vi "form voltage alarm string.vi"(0 "Xmon":dbl[][](array[numeric]), 1 "Xset":dbl[][](array[numeric]), 2 "Timestamps":dbl[][](array[numeric]), 3 "Alarm Tolerance (frac)":dbl=0.2 format="%#_13g", 4 "Warning Tolerance (frac)":dbl=0.1 format="%#_13g", 5 "error in":errorcluster, 6 "Alarm:T Warning:F":bool, 7 "Crate Enable":bool, 8 "Current:T Voltage:F":bool, 10 "Num Channels Read":i32, 12 "Start index":i32) -> (14 "Error Status String":string, 15 "All channels in error":string, 16 "Error Logged":bool[](array[boolean]), 17 "Error Array":string[][](array[string]), 18 "Status Strings":string[](array[string]), 19 "Error Out":errorcluster)   [LabVIEW 2018]
uses:
  channel_cluster.ctl
  CAEN globals.vi
  <userlib>/_OpenG.lib/array/array.llb/Search 1D Array (Boolean)__ogtk.vi
  <userlib>/_OpenG.lib/array/array.llb/Index 1D Array Elements (DBL)__ogtk.vi
  <userlib>/_OpenG.lib/array/array.llb/Index 1D Array Elements (Boolean)__ogtk.vi
  <userlib>/_OpenG.lib/array/array.llb/Index 1D Array Elements (String)__ogtk.vi
panel:
  in  "Channel Array Val":T1[](array[typedef]) {"Vfile (V)" format="%.1f V"}
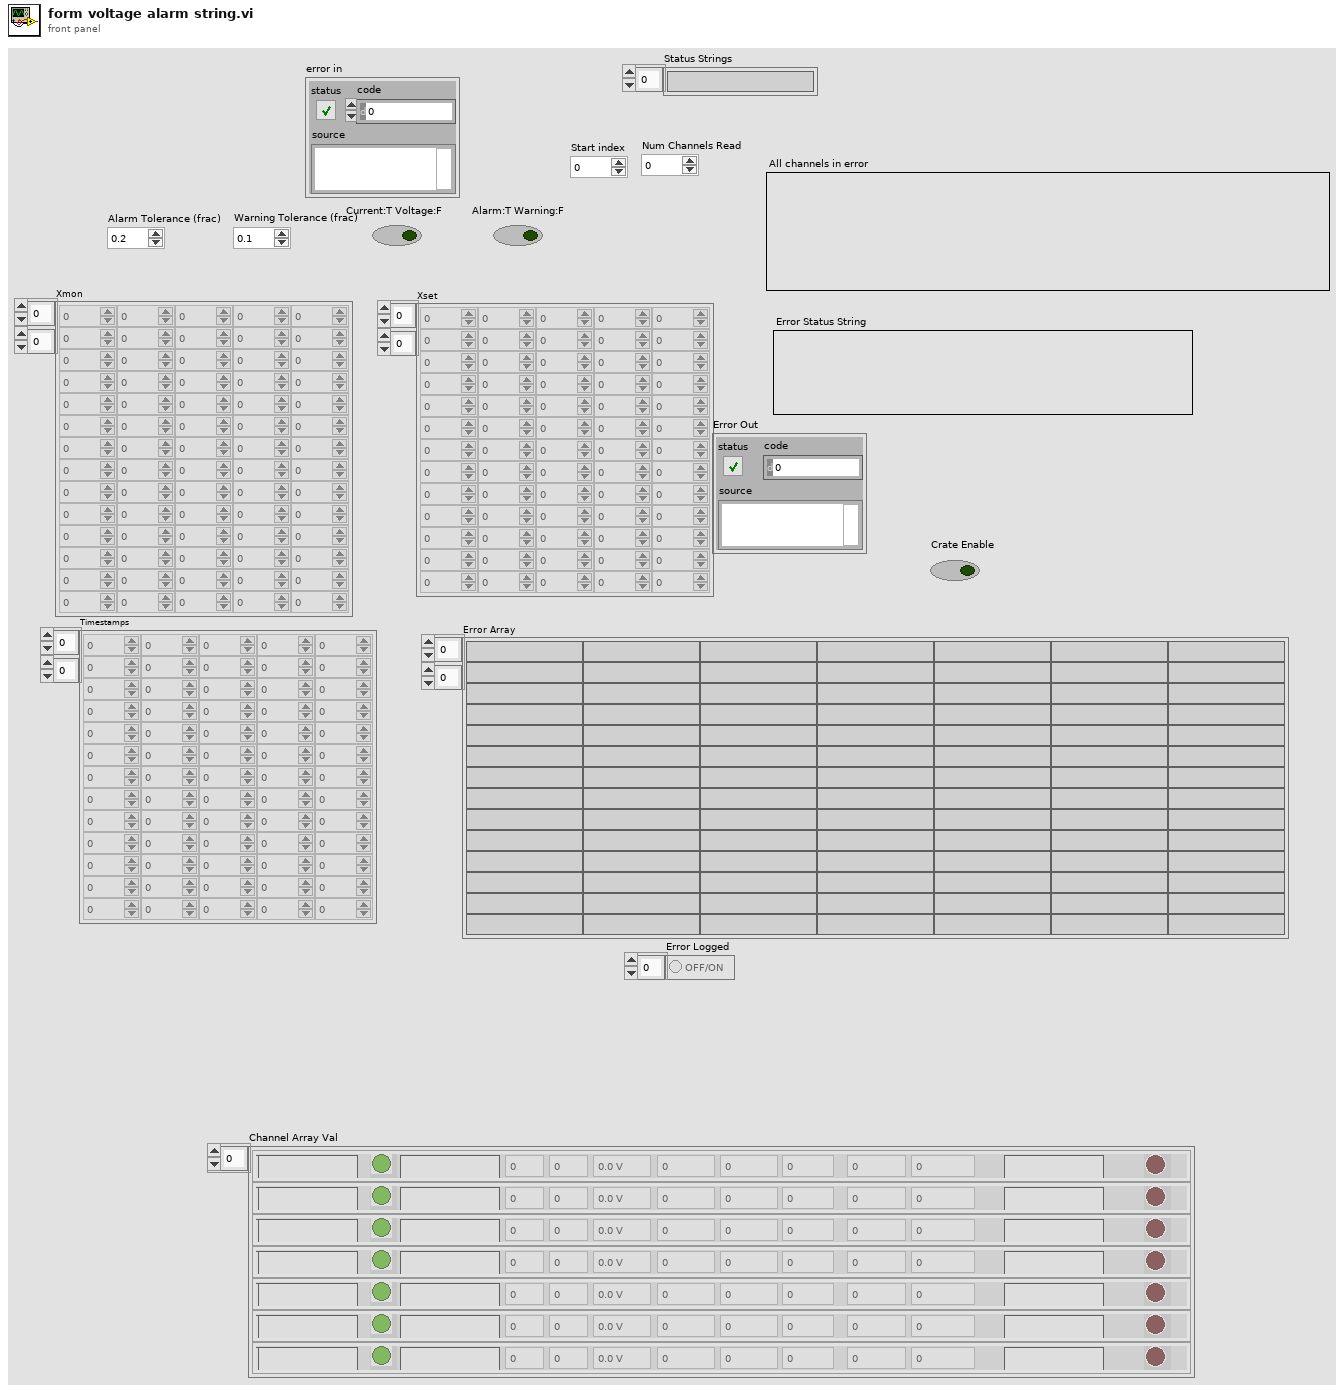
[diagram p1: front panel]
types:
  T1 = typedef "channel_cluster.ctl" = cluster{"Channel Name":string, "Crate":i32, "Card Type":string, "Card":i32, "Channel":i32, "Status Icon":picture, "Vmon (V)":dbl, "Vset (V)":dbl, "Imon (A)":dbl, "Iset (A)":dbl, "Timestamp":string, "ON/OFF":bool, "Status":string, "Vswmax (V)":dbl, "Flag":bool, "Vfile (V)":dbl, "Error Logged":bool[], "enable_file":bool}
  T2 = cluster{"Crate num":i32, "Slot nums":i32[], "Channel nums":i32[][], "N chans":i32[]}[]
  T3 = cluster{"Numeric":i32, "Indices of Elements":i32[], "Indices of Elements":i32[][], "Indices of Elements":i32[]}
  T4 = cluster{"Numeric":i32, "Indices of Elements":i32[], "Indices of Elements":i32[][], "Indices of Elements":i32[]}[]
  T5 = cluster{"Numeric":i32, "Indices of Elements":i32[], i32[][], i32[]}
  T6 = cluster{"Numeric":i32, "Indices of Elements":i32[], "Channel nums":i32[][], "N chans":i32[]}[]
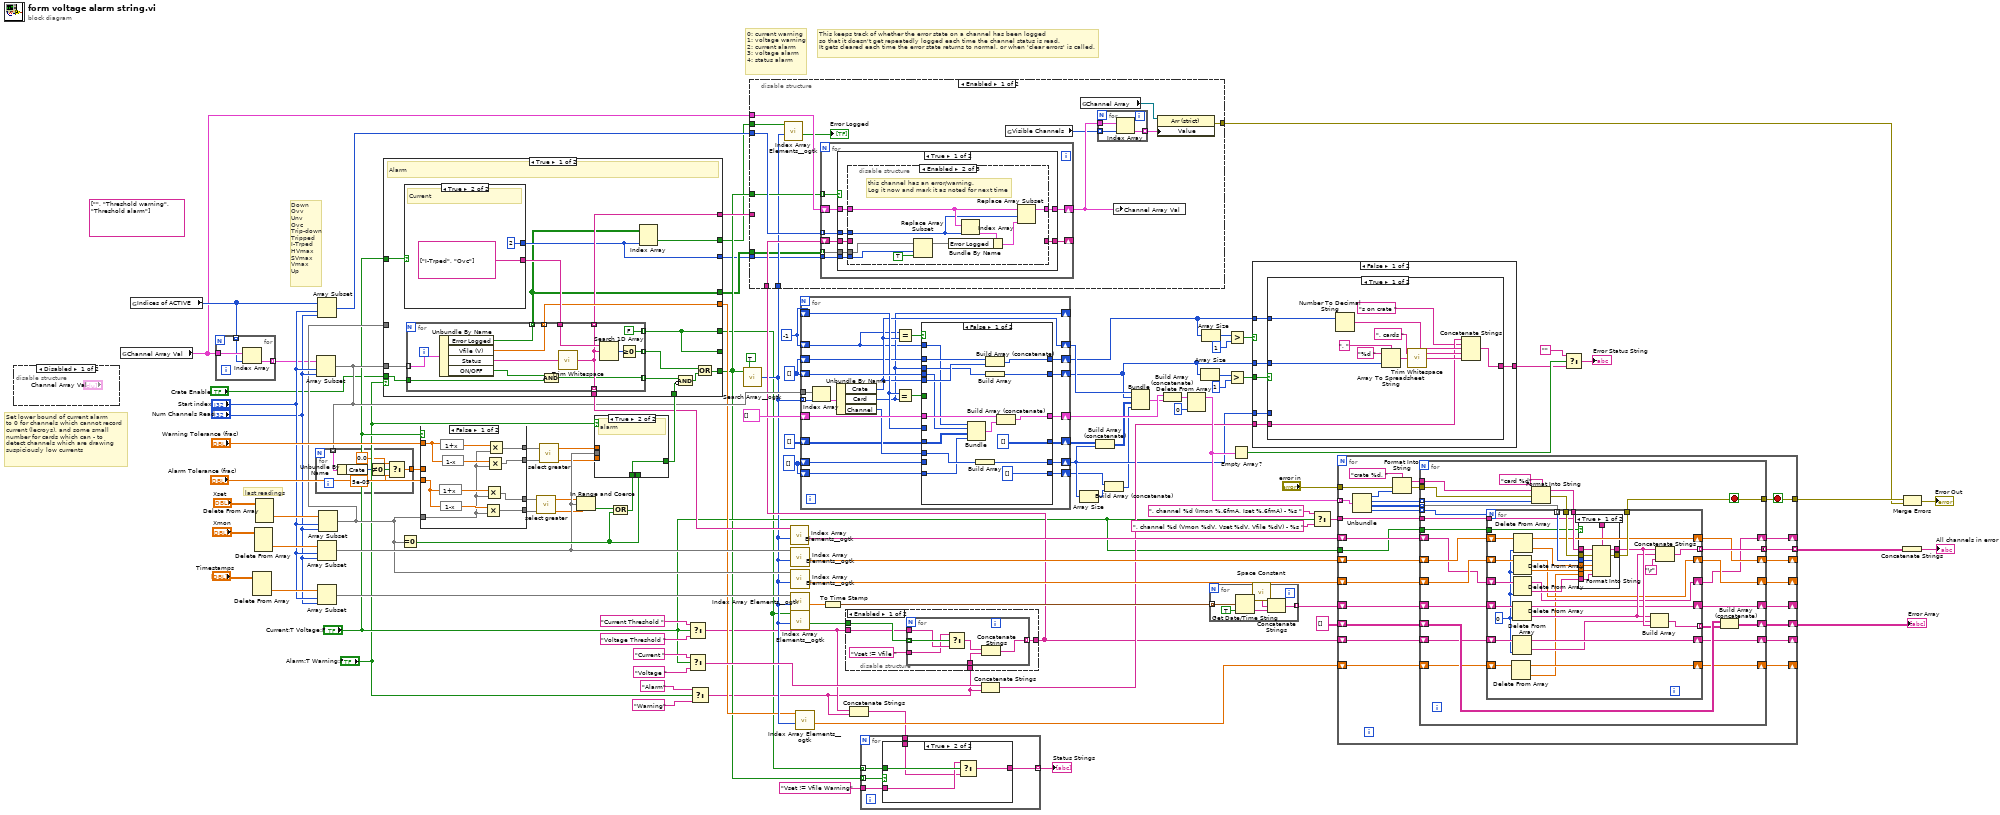
[diagram p0: block diagram]
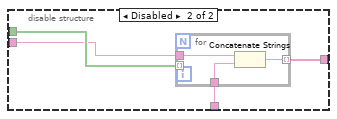
[diagram p2: hidden frame]
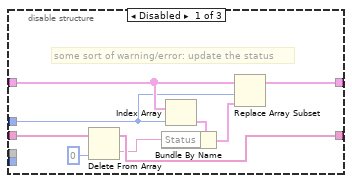
[diagram p3: hidden frame]
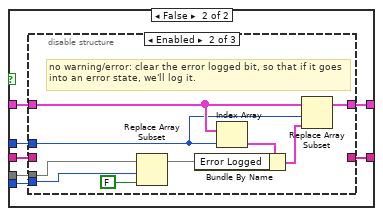
[diagram p5: hidden frame]
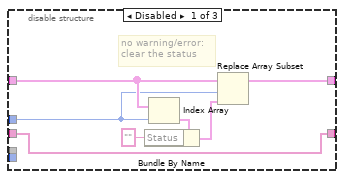
[diagram p6: hidden frame]
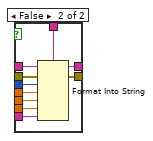
[diagram p11: hidden frame]
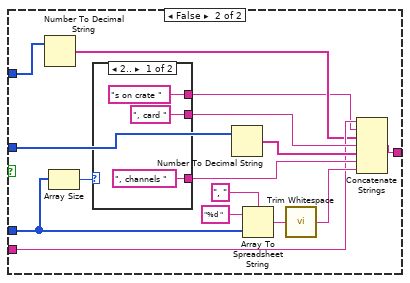
[diagram p12: hidden frame]
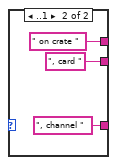
[diagram p13: hidden frame]
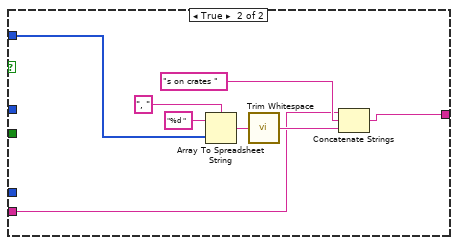
[diagram p14: hidden frame]
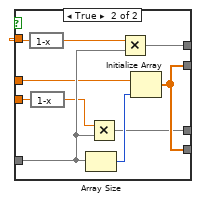
[diagram p15: hidden frame]
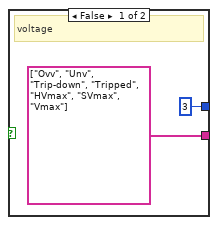
[diagram p16: hidden frame]
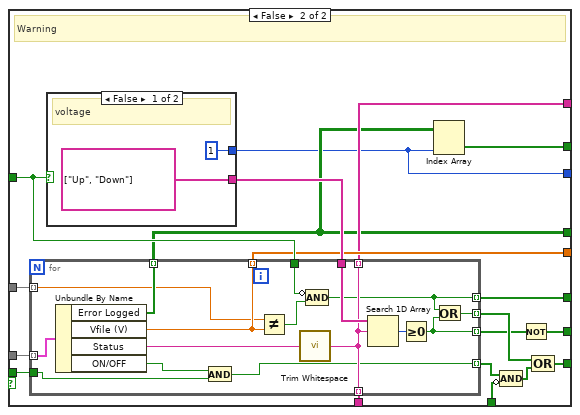
[diagram p17: hidden frame]
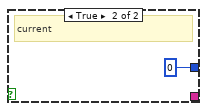
[diagram p18: hidden frame]
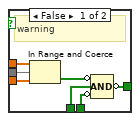
[diagram p19: hidden frame]
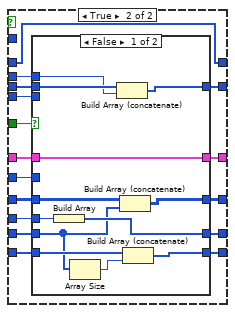
[diagram p20: hidden frame]
diagram:
  w33 = i32[] [] ("Indices of Elements")
  (unwired) string[] ["", "Threshold warning", "Threshold alarm"] ("items to filter")
  w45 = i32[] [] ("Indices of Elements")
  w46 = -1 ("Numeric")
  # "0: current warning\n1: voltage warning\n2: current alarm\n3: voltage alarm\n4: status alarm"
  # "This keeps track of whether the error state on a channel has been logged\nso that it doesn't get repeatedly logged each time the channel status is read.\nIt gets cleared each time the error state returns to normal, or when 'clear errors' is called."
  # "Set lower bound of current alarm\nto 0 for channels which cannot record\ncurrent (lecroys), and some small\nnumber for cards which can - to\ndetect channels which are drawing\nsuspiciously low currents"
  # "Down\nOvv\nUnv\nOvc\nTrip-down\nTripped\nI-Trped\nHVmax\nSVmax\nVmax\nUp"
  # "last readings"
  n1 = disable-structure shown="Disabled" {
    frame Disabled {
    }
    frame Enabled {
    }
  }
  n2 = global read "CAEN globals.vi" "Channel Array Val"() -> (w34:T1[])
  n3 = global read "CAEN globals.vi" "Indices of ACTIVE"() -> (w57:i32[])
  n4 = for {
    tunnel: w34 -> [w109]
    tunnel: [w108] -> w23 mode=indexing
    tunnel: w57 -> [w107] mode=indexing
    n5 = Index Array(array=w109, index=w107) -> (element=w108:T1)
  }
  n6 = Delete From Array(array="Timestamps") -> (deleted portion=w59:dbl[])  [unwired: 3 in, 1 out]
  n7 = Delete From Array(array="Xmon") -> (deleted portion=w61:dbl[])  [unwired: 3 in, 1 out]
  n8 = Delete From Array(array="Xset") -> (deleted portion=w62:dbl[])  [unwired: 3 in, 1 out]
  n9 = Array Subset(array=w23, index="Start index", length="Num Channels Read") -> (w52:T1[])
  n10 = for {
    tunnel: w52 -> [w115] mode=indexing
    tunnel: [w110] -> w51
    n11 = Unbundle By Name(w115) -> ("Crate"=w114:i32)
    n12 = Not Equal To 0?(x=w114) -> (x != 0?=w113:bool)
    n13 = Select(t=0.0 ("element"), s=w113, f=5e-05 ("element")) -> (s? t:f=w110:dbl)
  }
  n14 = Array Subset(array=w57, index="Start index", length="Num Channels Read") -> (w22:i32[])
  n15 = Array Subset(array=w61, index="Start index", length="Num Channels Read") -> (w60:dbl[])
  n16 = Array Subset(array=w59, index="Start index", length="Num Channels Read") -> (w58:dbl[])
  n17 = Array Subset(array=w62, index="Start index", length="Num Channels Read") -> (w35:dbl[])
  n18 = Equal To 0?(x=w35) -> (x = 0?=w72:bool[])
  n19 = case shown="False" "Current:T Voltage:F" {
    tunnel: [w118 w135] -> w11
    tunnel: [w119 w127] -> w14
    tunnel: [w124 w132] -> w10
    tunnel: [w122 w135] -> w9
    tunnel: "Warning Tolerance (frac)" -> [w126 w133]
    tunnel: "Alarm Tolerance (frac)" -> [w117 w131]
    tunnel: w35 -> [w116 w134]
    tunnel: w51 -> [_ w128]
    frame False {
      n20 = expression code="1+x"(w117) -> (w120:dbl)
      n21 = expression code="1+x"(w126) -> (w125:dbl)
      n22 = expression code="1-x"(w117) -> (w121:dbl)
      n23 = expression code="1-x"(w126) -> (w123:dbl)
      n24 = Multiply(x=w121, y=w116) -> (x*y=w118:dbl[])
      n25 = Multiply(x=w120, y=w116) -> (x*y=w119:dbl[])
      n26 = Multiply(x=w123, y=w116) -> (x*y=w122:dbl[])
      n27 = Multiply(x=w125, y=w116) -> (x*y=w124:dbl[])
    }
    frame True {
      n28 = expression code="1-x"(w133) -> (w130:dbl)
      n29 = expression code="1-x"(w131) -> (w129:dbl)
      n30 = Array Size(array=w134) -> (size(s)=w136:i32)
      n31 = Multiply(x=w129, y=w134) -> (x*y=w127:dbl[])
      n32 = Multiply(x=w130, y=w134) -> (x*y=w132:dbl[])
      n33 = Initialize Array(w128, w136) -> (w135:dbl[])
    }
  }
  n34 = call "select greater.vi"("Array 1 in"=w14, "Array 2 in"=w11) -> ("Array of higher vals"=w13:dbl[], "Array of lower vals"=w12:dbl[])  [unwired: 24 in]
  n35 = call "select greater.vi"("Array 1 in"=w10, "Array 2 in"=w9) -> ("Array of higher vals"=w7:dbl[], "Array of lower vals"=w8:dbl[])  [unwired: 24 in]
  n36 = In Range and Coerce(upper limit=w13, x=w60, lower limit=w12) -> (In Range?=w54:bool[])  [unwired: 1 out]
  n37 = Compound Arithmetic op=OR(w54, w72) -> (w65:bool[])
  n38 = case shown="True" "Alarm:T Warning:F" {
    tunnel: w60 -> [w143 _]
    tunnel: w65 -> [w137 w144]
    tunnel: [w141 w144] -> w74
    tunnel: w72 -> [w138 _]
    tunnel: w7 -> [w140 _]
    tunnel: w8 -> [w139 _]
    frame False {
      # "warning"
      n39 = In Range and Coerce(upper limit=w140, x=w143, lower limit=w139) -> (In Range?=w142:bool[])  [unwired: 1 out]
      n40 = Compound Arithmetic op=AND(invert w142, w137, invert w138) -> (invert w141:bool[])
    }
    frame True {
      # "alarm"
    }
  }
  n41 = case shown="True" "Alarm:T Warning:F" {
    tunnel: [w157 w192] -> w20
    tunnel: w74 -> [w156 w191]
    tunnel: [w160 w195] -> w73
    tunnel: [w151 w184] -> w21
    tunnel: w52 -> [w159 w194]
    tunnel: "Current:T Voltage:F" -> [w153 w186]
    tunnel: [w145 w179] -> _
    tunnel: w35 -> [_ w187]
    tunnel: [w152 w185] -> w26
    tunnel: [w150 w183] -> w6
    tunnel: [w148 w182] -> w5
    tunnel: [w149 w181] -> w4
    tunnel: "Crate Enable" -> [w146 w178]
    tunnel: [w145 w177] -> w1
    frame True {
      # "Alarm"
      n42 = case shown="True" w153 {
        tunnel: [string[] ["Ovv", "Unv", "Trip-down", "Tripped", "HVmax", "SVmax", "Vmax"] ("items to filter") string[] ["I-Trped", "Ovc"] ("items to filter")] -> w154
        tunnel: [3 2] -> w149
        frame False {
          # "voltage"
        }
        frame True {
          # "Current"
        }
      }
      n43 = for {
        tunnel: w159 -> [w176] mode=indexing
        tunnel: [w171] -> w158 mode=indexing
        tunnel: w154 -> [w174]
        tunnel: [w172] -> w160 mode=indexing
        tunnel: [w172] -> w151 mode=indexing
        tunnel: [FALSE ("Element Data")] -> w145 mode=indexing
        tunnel: [w169] -> w152 mode=indexing
        tunnel: [w168] -> w148 mode=indexing
        tunnel: [w166] -> w147 mode=indexing
        tunnel: w146 -> [w165]
        n44 = Unbundle By Name(w176) -> ("Error Logged"=w168:bool[], "Vfile (V)"=w169:dbl, "Status"=w173:string, "ON/OFF"=w167:bool)
        n45 = And(x=w167, y=w165) -> (x .and. y?=w166:bool)
        n46 = call <vilib>:"Trim Whitespace.vi"("string"=w173) -> ("trimmed string"=w172:string)  [unwired: 1 in]
        n47 = Search 1D Array(1D array=w174, element=w172) -> (index of element=w175:i32)  [unwired: 1 in]
        n48 = Greater Or Equal To 0?(x=w175) -> (x >= 0?=w171:bool)
      }
      n49 = Index Array(array=w148, index (col)=w149) -> (element=w150:bool[])  [unwired: 1 in]
      n50 = Compound Arithmetic op=AND(w147, invert w156) -> (w155:bool[])
      n51 = Compound Arithmetic op=OR(w158, w155) -> (w157:bool[])
    }
    frame False {
      # "Warning"
      n52 = case shown="False" w186 {
        tunnel: [string[] ["Up", "Down"] ("items to filter") _] -> w188
        tunnel: [1 0] -> w181
        frame False {
          # "voltage"
        }
        frame True {
          # "current"
        }
      }
      n53 = for {
        tunnel: w194 -> [w214] mode=indexing
        tunnel: [w201] -> w190 mode=indexing
        tunnel: [w205] -> w193 mode=indexing
        tunnel: w188 -> [w212]
        tunnel: [w210] -> w195 mode=indexing
        tunnel: [w210] -> w184 mode=indexing
        tunnel: w187 -> [w203] mode=indexing
        tunnel: w186 -> [w208]
        tunnel: [w207] -> w185 mode=indexing
        tunnel: [w206] -> w182 mode=indexing
        tunnel: [w204] -> w180 mode=indexing
        tunnel: w178 -> [w200]
        tunnel: [w199] -> w177 mode=indexing
        n54 = Unbundle By Name(w214) -> ("Error Logged"=w206:bool[], "Vfile (V)"=w207:dbl, "Status"=w211:string, "ON/OFF"=w202:bool)
        n55 = And(x=w202, y=w200) -> (x .and. y?=w201:bool)
        n56 = Not Equal?(x=w203, y=w207) -> (x != y?=w209:bool)
        n57 = call <vilib>:"Trim Whitespace.vi"("string"=w211) -> ("trimmed string"=w210:string)  [unwired: 1 in]
        n58 = Compound Arithmetic op=AND(invert w208, w209) -> (w199:bool)
        n59 = Search 1D Array(1D array=w212, element=w210) -> (index of element=w213:i32)  [unwired: 1 in]
        n60 = Greater Or Equal To 0?(x=w213) -> (x >= 0?=w204:bool)
        n61 = Or(x=w199, y=w204) -> (x .or. y?=w205:bool)
      }
      n62 = Index Array(array=w182, index (col)=w181) -> (element=w183:bool[])  [unwired: 1 in]
      n63 = Compound Arithmetic op=AND(w190, invert w191) -> (w189:bool[])
      n64 = Not(x=w180) -> (.not. x?=w179:bool[])
      n65 = Compound Arithmetic op=OR(w193, w189) -> (w192:bool[])
    }
  }
  n66 = Select(t="Current Threshold " ("Card type"), s="Current:T Voltage:F", f="Voltage Threshold " ("Card type")) -> (s? t:f=w18:string)
  n67 = Select(t="Current " ("Card type"), s="Current:T Voltage:F", f="Voltage " ("Card type")) -> (s? t:f=w47:string)
  n68 = Select(t="Alarm" ("Card type"), s="Alarm:T Warning:F", f="Warning" ("Card type")) -> (s? t:f=w17:string)
  n69 = call-poly <userlib>:"Search Array__ogtk.vi"("Array"=w20, "Element Data"=TRUE) -> ("Indices of Elements"=w27:i32[])  [unwired: 7 in]
  n70 = call-poly <userlib>:"Index Array Elements__ogtk.vi"("indices"=w27, "array"=w73) -> ("elements"=w55:string[])  [unwired: 9 in]
  n71 = call-poly <userlib>:"Index Array Elements__ogtk.vi"("indices"=w27, "array"=w60) -> ("elements"=w80:dbl[])  [unwired: 9 in]
  n72 = call-poly <userlib>:"Index Array Elements__ogtk.vi"("indices"=w27, "array"=w35) -> ("elements"=w79:dbl[])  [unwired: 9 in]
  n73 = call-poly <userlib>:"Index Array Elements__ogtk.vi"("indices"=w27, "array"=w58) -> ("elements"=w75:dbl[])  [unwired: 9 in]
  n74 = call-poly <userlib>:"Index Array Elements__ogtk.vi"("indices"=w27, "array"=w1) -> ("elements"=w28:bool[])  [unwired: 9 in]
  n75 = call-poly <userlib>:"Index Array Elements__ogtk.vi"("indices"=w27, "array"=w26) -> ("elements"=w25:dbl[])  [unwired: 9 in]
  n76 = for {
    tunnel: w27 -> [w231] mode=indexing
    shift-right: [w221] -> _
    shift-left: w46 -> [w227]
    shift-right: [w236] -> w40
    shift-left: i32[][] [] ("Indices of Elements") -> [w217]
    shift-right: [w235] -> w91
    shift-left: T2 [] -> [w234]
    shift-right: [w232] -> w37
    shift-left: w45 -> [w233]
    tunnel: w52 -> [w230]
    shift-right: [w224] -> w42
    shift-left: w46 -> [w220]
    shift-right: [w222] -> w38
    shift-left: w45 -> [w223]
    shift-right: [w218] -> w32
    shift-left: w33 -> [w219]
    shift-right: [w215] -> w30
    shift-left: w33 -> [w216]
    n77 = Index Array(array=w230, index=w231) -> (element=w229:T1)
    n78 = Unbundle By Name(w229) -> ("Crate"=w224:i32, "Card"=w221:i32, "Channel"=w228:i32)
    n79 = Equal?(x=w227, y=w221) -> (x = y?=w225:bool)
    n80 = Equal?(x=w220, y=w224) -> (x = y?=w226:bool)
    n81 = case shown="False" w226 {
      tunnel: w217 -> [w241 w268]
      tunnel: [i32[][] [] ("Indices of Elements") w267] -> w236
      tunnel: [w248 w266] -> w235
      tunnel: w234 -> [w249 w265]
      tunnel: w233 -> [w242 w264]
      tunnel: [w244 w263] -> w232
      tunnel: w228 -> [w246 w262]
      tunnel: w227 -> [_ w261]
      tunnel: w225 -> [_ w260]
      tunnel: w224 -> [w247 w259]
      tunnel: w223 -> [w252 w258]
      tunnel: [w251 w258] -> w222
      tunnel: w221 -> [w245 w255]
      tunnel: w220 -> [w243 _]
      tunnel: w219 -> [_ w256]
      tunnel: [w240 w257] -> w218
      tunnel: w216 -> [w238 w254]
      tunnel: [i32[] [] ("Indices of Elements") w253] -> w215
      frame False {
        n82 = Bundle("Numeric"=w243, "Indices of Elements"=w242, "Indices of Elements"=w241, "Indices of Elements"=w238) -> (w250:T3)  [unwired: 1 in]
        n83 = Build Array(w246) -> (w240:i32[])
        n84 = Build Array (concatenate)(w252, w247) -> (w251:i32[])
        n85 = Build Array(w245) -> (w244:i32[])
        n86 = Build Array (concatenate)(w249, w250) -> (w248:T4)
      }
      frame True {
        n87 = case shown="False" w260 {
          tunnel: w268 -> [w274 w285]
          tunnel: w262 -> [w277 w283]
          tunnel: [w280 w285] -> w267
          tunnel: [w276 w287] -> w266
          tunnel: w265 -> [w276 w287]
          tunnel: w261 -> [_ _]
          tunnel: w264 -> [w278 w286]
          tunnel: [w279 w286] -> w263
          tunnel: w259 -> [_ _]
          tunnel: [w275 w282] -> w257
          tunnel: w256 -> [w269 w284]
          tunnel: w255 -> [w273 _]
          tunnel: w254 -> [w272 w281]
          tunnel: [w271 w281] -> w253
          frame False {
            n88 = Build Array(w277) -> (w275:i32[])
            n89 = Array Size(array=w269) -> (size(s)=w270:i32)
            n90 = Build Array (concatenate)(w278, w273) -> (w279:i32[])
            n91 = Build Array (concatenate)(w274, w269) -> (w280:i32[][])
            n92 = Build Array (concatenate)(w272, w270) -> (w271:i32[])
          }
          frame True {
            n93 = Build Array (concatenate)(w284, w283) -> (w282:i32[])
          }
        }
      }
    }
  }
  n94 = To Time Stamp(1:w75) -> (0:w64:timestamp[])
  n95 = disable-structure shown="Enabled" {
    disable-tunnel: [w292 w302] -> w36
    disable-tunnel: w28 -> [w291 w301]
    disable-tunnel: w18 -> [w289 w300]
    disable-tunnel: w17 -> [w288 w299]
    frame Enabled {
      n96 = for {
        tunnel: w289 -> [w297]
        tunnel: w291 -> [w298] mode=indexing
        tunnel: "Vset != Vfile " ("Card type") -> [w296]
        tunnel: [w293] -> w292 mode=indexing
        tunnel: w288 -> [w295]
        n97 = Select(t=w296, s=w298, f=w297) -> (s? t:f=w294:string)
        n98 = Concatenate Strings(w294, w295) -> (w293:string)
      }
    }
    frame Disabled {
      n99 = for {
        tunnel: w300 -> [w303]
        tunnel: w301 -> [_] mode=indexing
        tunnel: [w304] -> w302 mode=indexing
        tunnel: w299 -> [w305]
        n100 = Concatenate Strings(w303, w305) -> (w304:string)
      }
    }
  }
  n101 = disable-structure shown="Enabled" {
    disable-tunnel: [w319 _] -> w67
    disable-tunnel: w36 -> [w314 _]
    disable-tunnel: w34 -> [w313 _]
    disable-tunnel: w27 -> [w310 _]
    disable-tunnel: w22 -> [w312 _]
    disable-tunnel: w21 -> [_ _]
    disable-tunnel: w20 -> [w311 _]
    disable-tunnel: w6 -> [w308 _]
    disable-tunnel: w5 -> [w307 _]
    disable-tunnel: w4 -> [w306 _]
    frame Enabled {
      n102 = call-poly <userlib>:"Index Array Elements__ogtk.vi"("indices"=w310, "array"=w308) -> ("elements"=→"Error Logged":bool[])  [unwired: 9 in]
      n103 = for {
        shift-right: [w328] -> w318
        shift-left: w313 -> [w330]
        tunnel: w312 -> [w329] mode=indexing
        tunnel: w311 -> [w326] mode=indexing
        shift-right: [w325] -> _
        shift-left: w314 -> [w327]
        tunnel: w307 -> [w324] mode=indexing
        tunnel: w306 -> [w323]
        n104 = case shown="True" w326 {
          tunnel: w330 -> [w337 w362]
          tunnel: w329 -> [w336 w361]
          tunnel: [w335 w360] -> w328
          tunnel: w327 -> [w334 w359]
          tunnel: [w333 w358] -> w325
          tunnel: w324 -> [w332 w357]
          tunnel: w323 -> [w331 w356]
          frame True {
            n105 = disable-structure shown="Enabled" {
              disable-tunnel: w337 -> [w346 w355 _]
              disable-tunnel: w336 -> [w345 w354 _]
              disable-tunnel: [w344 w353 _] -> w335
              disable-tunnel: w334 -> [w343 _ _]
              disable-tunnel: [w342 _ _] -> w333
              disable-tunnel: w332 -> [_ w350 _]
              disable-tunnel: w331 -> [_ w349 _]
              frame Disabled {
                # "some sort of warning/error: update the status"
                n106 = Delete From Array(array=w343, index=0) -> (deleted portion=w340:string, array with subset deleted=w342:string[])  [unwired: 1 in]
                n107 = Index Array(array=w346, index=w345) -> (element=w339:T1)
                n108 = Bundle By Name(cluster=w339, "Status"=w340) -> (w338:T1)
                n109 = Replace Array Subset(array=w346, new element=w338, index=w345) -> (w344:T1[])
              }
              frame Enabled {
                # "this channel has an error/warning. \nLog it now and mark it as noted for next time"
                n110 = Replace Array Subset(array=w350, new element=TRUE ("Element Data"), index=w349) -> (w348:bool[])
                n111 = Index Array(array=w355, index=w354) -> (element=w352:T1)
                n112 = Bundle By Name(cluster=w352, "Error Logged"=w348) -> (w351:T1)
                n113 = Replace Array Subset(array=w355, new element=w351, index=w354) -> (w353:T1[])
              }
              frame Disabled {
              }
            }
          }
          frame False {
            n114 = disable-structure shown="Enabled" {
              disable-tunnel: w362 -> [w369 w378 _]
              disable-tunnel: w361 -> [w368 w377 _]
              disable-tunnel: [w367 w376 _] -> w360
              disable-tunnel: [w363 _ _] -> w358
              disable-tunnel: w359 -> [w363 _ _]
              disable-tunnel: w357 -> [_ w372 _]
              disable-tunnel: w356 -> [_ w371 _]
              frame Disabled {
                # "no warning/error:\nclear the status"
                n115 = Index Array(array=w369, index=w368) -> (element=w366:T1)
                n116 = Bundle By Name(cluster=w366, "Status"="") -> (w365:T1)
                n117 = Replace Array Subset(array=w369, new element=w365, index=w368) -> (w367:T1[])
              }
              frame Enabled {
                # "no warning/error: clear the error logged bit, so that if it goes into an error state, we'll log it."
                n118 = Replace Array Subset(array=w372, new element=FALSE ("Element Data"), index=w371) -> (w373:bool[])
                n119 = Index Array(array=w378, index=w377) -> (element=w375:T1)
                n120 = Bundle By Name(cluster=w375, "Error Logged"=w373) -> (w374:T1)
                n121 = Replace Array Subset(array=w378, new element=w374, index=w377) -> (w376:T1[])
              }
              frame Disabled {
              }
            }
          }
        }
      }
      n122 = global read "CAEN globals.vi" "Visible Channels"() -> (w317:i32[])
      n123 = global read "CAEN globals.vi" "Channel Array"() -> (w316:refnum<vi>)
      n124 = for {
        tunnel: w318 -> [w322]
        tunnel: w317 -> [w321] mode=indexing
        tunnel: [w320] -> w315 mode=indexing
        n125 = Index Array(array=w322, index=w321) -> (element=w320:T1)
      }
      n126 = global write "CAEN globals.vi" "Channel Array Val"(w318) -> ()
      n127 = property class="Arr (strict)"(reference=w316, "Value"=w315) -> (error out=w319:errorcluster)  [unwired: 1 in, 1 out]
    }
    frame Disabled {
    }
  }
  n128 = Concatenate Strings(w18, w17) -> (w16:string)
  n129 = for {
    tunnel: w1 -> [w382] mode=indexing
    tunnel: w20 -> [w383] mode=indexing
    tunnel: "Vset != Vfile Warning" ("Card type") -> [w381]
    tunnel: w16 -> [w380]
    tunnel: [w379] -> w15 mode=indexing
    n130 = case shown="True" w383 {
      tunnel: w382 -> [_ w387]
      tunnel: w381 -> [_ w386]
      tunnel: w380 -> [_ w385]
      tunnel: [_ w384] -> w379
      frame False {
      }
      frame True {
        n131 = Select(t=w386, s=w387, f=w385) -> (s? t:f=w384:string)
      }
    }
  }
  "Status Strings" <- w15
  n132 = Concatenate Strings(w47, w17) -> (w53:string)
  n133 = Array Size(array=w32) -> (size(s)=w31:i32)
  n134 = Build Array (concatenate)(w40, w32) -> (w39:i32[][])
  n135 = Build Array (concatenate)(w30, w31) -> (w29:i32[])
  n136 = Bundle("Numeric"=w42, "Indices of Elements"=w37, w39, w29) -> (w90:T5)  [unwired: 1 in]
  n137 = Build Array (concatenate)(w91, w90) -> (w89:T6)
  n138 = Delete From Array(array=w89, index=0) -> (array with subset deleted=w88:T6)  [unwired: 1 in, 1 out]
  n139 = Array Size(array=w37) -> (size(s)=w103:i32)
  n140 = Array Size(array=w38) -> (size(s)=w43:i32)
  n141 = for {
    tunnel: w64 -> [w389] mode=indexing
    tunnel: [w388] -> w63 mode=indexing
    n142 = Get Date/Time String(seconds (now)=w389, want seconds? (F)=TRUE) -> (date string=w392:string, time string=w390:string)  [unwired: 1 in]
    n143 = call <vilib>:"Space Constant.vi"() -> ("String"=w393:string)
    n144 = Concatenate Strings(w392, w393, w390) -> (w388:string)
  }
  n145 = Greater?(x=w103, y=1) -> (0:w101:bool)
  n146 = Greater?(x=w43, y=1) -> (0:w41:bool)
  n147 = Empty Array?(array=w88) -> (empty?=w106:bool)
  n148 = case shown="False" w41 {
    tunnel: w101 -> [w399 _]
    tunnel: w32 -> [w398 _]
    tunnel: w37 -> [w397 _]
    tunnel: [w396 w434] -> w78
    tunnel: w53 -> [w395 w433]
    tunnel: w38 -> [w394 w432]
    frame False {
      n149 = case shown="True" w399 {
        tunnel: w397 -> [w405 w424]
        tunnel: [w409 w425] -> w396
        tunnel: w398 -> [_ w423]
        tunnel: w395 -> [w401 w414]
        tunnel: w394 -> [w402 w412]
        frame True {
          n150 = Number To Decimal String(number=w402) -> (decimal integer string=w403:string[])  [unwired: 1 in]
          n151 = Array To Spreadsheet String(delimiter (Tab)=", ", array=w405, 3:"%d " ("delimiter (Tab)")) -> (spreadsheet string=w407:string)
          n152 = call <vilib>:"Trim Whitespace.vi"("string"=w407) -> ("trimmed string"=w406:string)  [unwired: 1 in]
          n153 = Concatenate Strings(w401, "s on crate " ("Card type"), w403, ", cards " ("Card type"), w406) -> (w409:string)
        }
        frame False {
          n154 = Number To Decimal String(number=w412) -> (decimal integer string=w413:string[])  [unwired: 1 in]
          n155 = Array Size(array=w423) -> (size(s)=w417:i32)
          n156 = case shown="2.." w417 {
            tunnel: [", channels " ("Card type") ", channel " ("Card type")] -> w416
            tunnel: [", card " ("Card type") ", card " ("Card type")] -> w415
            tunnel: ["s on crate " ("Card type") " on crate " ("Card type")] -> w411
            frame 2.. {
            }
            frame ..1 {
            }
          }
          n157 = Number To Decimal String(number=w424) -> (decimal integer string=w419:string[])  [unwired: 1 in]
          n158 = Array To Spreadsheet String(delimiter (Tab)=", ", array=w423, 3:"%d " ("delimiter (Tab)")) -> (spreadsheet string=w421:string)
          n159 = call <vilib>:"Trim Whitespace.vi"("string"=w421) -> ("trimmed string"=w420:string)  [unwired: 1 in]
          n160 = Concatenate Strings(w414, w411, w413, w415, w419, w416, w420) -> (w425:string)
        }
      }
    }
    frame True {
      n161 = Array To Spreadsheet String(delimiter (Tab)=", ", array=w432, 3:"%d " ("delimiter (Tab)")) -> (spreadsheet string=w439:string)
      n162 = call <vilib>:"Trim Whitespace.vi"("string"=w439) -> ("trimmed string"=w438:string)  [unwired: 1 in]
      n163 = Concatenate Strings(w433, "s on crates " ("Card type"), w438) -> (w434:string)
    }
  }
  n164 = Select(t=", channel %d (Imon %.6fmA, Iset %.6fmA) - %s " ("delimiter (Tab)"), s="Current:T Voltage:F", f=", channel %d (Vmon %dV, Vset %dV, Vfile %dV) - %s " ("delimiter (Tab)")) -> (s? t:f=w76:string)
  n165 = for {
    tunnel: [w466] -> w98 mode=indexing
    tunnel: w88 -> [w460] mode=indexing
    tunnel: w76 -> [w463]
    tunnel: "error in" -> [w459]
    tunnel: [w461] -> w69
    shift-right: [w464] -> w95
    shift-left: string[][] [] -> [w465]
    shift-right: [w447] -> _
    shift-left: w55 -> [w454]
    shift-right: [w444] -> _
    shift-left: w80 -> [w453]
    shift-right: [w445] -> _
    shift-left: w79 -> [w452]
    shift-right: [w448] -> _
    shift-left: w63 -> [w451]
    shift-right: [w446] -> _
    shift-left: w36 -> [w462]
    shift-right: [w441] -> _
    shift-left: w25 -> [w442]
    tunnel: "Current:T Voltage:F" -> [w440]
    stop <- w461 stop-if-true
    n166 = Unbundle(w460) -> ("Numeric"=w456:i32, "Indices of Elements"=w450:i32[], "Channel nums"=w449:i32[][], "N chans"=w443:i32[])
    n167 = Format Into String(format string="crate %d, " ("Card type"), error in=w459, w456) -> (resulting string=w455:string, error out=w458:errorcluster)  [unwired: 1 in]
    n168 = for {
      tunnel: w463 -> [w468]
      tunnel: [w492] -> w466 mode=concatenating
      shift-right: [w491] -> w464
      shift-left: w465 -> [w490]
      tunnel: w458 -> [w487]
      tunnel: [w485] -> w461
      tunnel: w450 -> [w484] mode=indexing
      tunnel: w449 -> [w472] mode=indexing
      tunnel: w455 -> [w483]
      shift-right: [w478] -> w448
      shift-left: w451 -> [w480]
      shift-right: [w476] -> w445
      shift-left: w452 -> [w481]
      shift-right: [w477] -> w444
      shift-left: w453 -> [w482]
      shift-right: [w475] -> w447
      shift-left: w454 -> [w479]
      shift-right: [w473] -> w446
      shift-left: w462 -> [w474]
      tunnel: w443 -> [w471] mode=indexing
      shift-right: [w469] -> w441
      shift-left: w442 -> [w470]
      tunnel: w440 -> [w467]
      stop <- w485 stop-if-true
      n169 = Format Into String(format string="card %d" ("Card type"), initial string=w483, error in=w487, w484) -> (resulting string=w493:string, error out=w486:errorcluster)
      n170 = for {
        N: w471 -> [_]
        tunnel: w472 -> [w519] mode=indexing
        tunnel: w493 -> [w522]
        tunnel: [w515] -> w492 mode=indexing
        tunnel: [w521] -> w485
        tunnel: [w520] -> w489 mode=indexing
        tunnel: w486 -> [w518]
        shift-right: [w512] -> w478
        shift-left: w480 -> [w514]
        shift-right: [w503] -> w477
        shift-left: w482 -> [w509]
        shift-right: [w504] -> w476
        shift-left: w481 -> [w507]
        shift-right: [w505] -> w475
        shift-left: w479 -> [w511]
        shift-right: [w500] -> w473
        shift-left: w474 -> [w502]
        shift-right: [w497] -> w469
        shift-left: w470 -> [w498]
        tunnel: w468 -> [w495]
        tunnel: w467 -> [w494]
        w501 = 0 ("index")
        n171 = Delete From Array(array=w498) -> (deleted portion=w496:dbl, array with subset deleted=w497:dbl[])  [unwired: 2 in]
        n172 = Delete From Array(array=w514, index=w501) -> (deleted portion=w513:string, array with subset deleted=w512:string[])  [unwired: 1 in]
        n173 = Delete From Array(array=w502, index=w501) -> (deleted portion=w499:string, array with subset deleted=w500:string[])  [unwired: 1 in]
        n174 = Delete From Array(array=w507, index=w501) -> (deleted portion=w506:dbl, array with subset deleted=w504:dbl[])  [unwired: 1 in]
        n175 = Delete From Array(array=w511, index=w501) -> (deleted portion=w510:string, array with subset deleted=w505:string[])  [unwired: 1 in]
        n176 = Delete From Array(array=w509, index=w501) -> (deleted portion=w508:dbl, array with subset deleted=w503:dbl[])  [unwired: 1 in]
        n177 = case shown="True" w494 {
          tunnel: w522 -> [w531 w541]
          tunnel: [w530 w540] -> w521
          tunnel: w519 -> [w529 w539]
          tunnel: w518 -> [w528 w538]
          tunnel: [w527 w537] -> w517
          tunnel: w510 -> [w526 w536]
          tunnel: w508 -> [w525 w535]
          tunnel: w506 -> [w524 w534]
          tunnel: w496 -> [_ w533]
          tunnel: w495 -> [w523 w532]
          frame True {
            n178 = Format Into String(format string=w523, initial string=w531, error in=w528, w529, w525, w524, w526) -> (resulting string=w527:string, error out=w530:errorcluster)
          }
          frame False {
            n179 = Format Into String(format string=w532, initial string=w541, error in=w538, w539, w535, w534, w533, w536) -> (resulting string=w537:string, error out=w540:errorcluster)
          }
        }
        n180 = Build Array(w513, w499, w517) -> (w520:string[])
        n181 = Concatenate Strings(w517, w513, "\r") -> (w515:string)
      }
      n182 = Build Array (concatenate)(w490, w489) -> (w491:string[][])
    }
  }
  "Error Array" <- w95
  n183 = Select(t="", s=w106, f=w78) -> (s? t:f=→"Error Status String":string)
  n184 = Concatenate Strings(w98) -> (→"All channels in error":string)
  n185 = Merge Errors(w69, w67) -> (→"Error Out":errorcluster)
